vi "Actor Core.vi"(8 "error in":errorcluster, 11 "Bottom Panel in":refnum<class "BottomDock.lvclass">) -> (0 "error out":errorcluster, 3 "Actor out":refnum<class "Actor.lvclass">)   [LabVIEW 2023, in "Docking.lvlib" / "BottomDock.lvclass"]
doc: "Base Class for the bottom subpanel.\nThis provides the basic implementation for show/hide operations.\n\nancestor classes should override this, but maintain proportions."
uses:
  BottomDock.lvclass
  builds/Framework/Actor Framework.lvlibp/1abvi3w/vi.lib/ActorFramework/Actor/Actor.lvclass
  Docking/Docking.lvclass
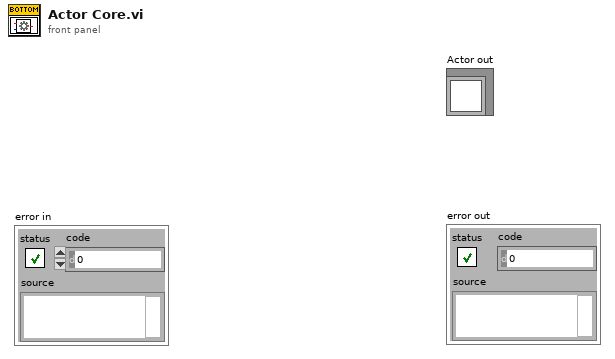
[diagram p1: front panel]
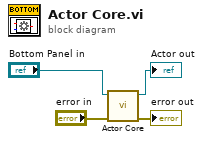
[diagram p0: block diagram]
diagram:
  n1 = call-parent "Actor Core.vi"("error in"="error in", "Panel Actor in"="Bottom Panel in") -> ("error out"=→"error out":errorcluster, "Actor out"=→"Actor out":refnum<class "Actor.lvclass">)  [unwired: 8 in]
